vi "Scan Engine.vi"(6 "Message Packet":T1={"Message"="Init", "Parameter"=variant}, 8 "Error In":errorcluster) -> (0 "Error Out":errorcluster)   [LabVIEW 2018]
uses:
  Controls/MessagePacket.ctl
  Controls/QueueNames.ctl
  Controls/Queue Manager Actions.ctl
  Controls/Go Scan Actions.ctl
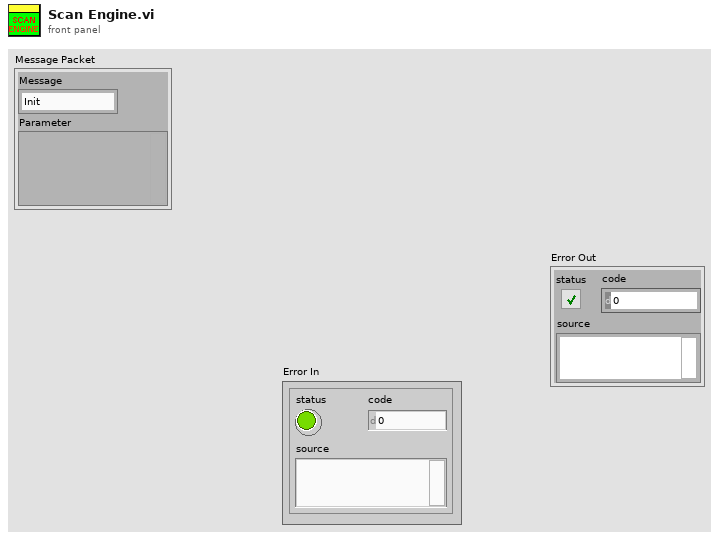
[diagram p1: front panel]
types:
  T1 = typedef "MessagePacket.ctl" = cluster{"Message":string, "Parameter":variant}
  T2 = typedef "Queue Manager Actions.ctl" = enum16{"Init", "Enqueue", "Enqueue All", "Preview Queue", "Dequeue", "Get Status", "Flush Queue", "Flush All Queues", "Release All Queues", "Release Queue", "Enqueue at Opposite End"}
  T3 = typedef "QueueNames.ctl" = enum16{"Main GUI", "Main Scan Processor", "Main Processing", "Main Saving", "Main Display", "Main Table Stage GUI", "Main Table Stage Proc.", "Scan Engine", "Vibratome GUI", "Vibratome Processor", "Slice Engine"}
  T4 = typedef "Go Scan Actions.ctl" = enum16{"Init(ThorOCT Spatial)", "Init(ThorOCT Spectral)", "Init(GPU FFT)", "Init(Alazar FFT)", "Init Scan Head(ThorOCT Spectral)", "Init Scan Head(ThorOCT Spatial)", "Init Scan Head", "Init Table Stage", "Init Vibratome", "Generate Mosaic", "Generate Z Position", "Go to Image Z", "Go Image Home", "Go Mosaic", "Acquire Image(ThorOCT Spatial)", "Acquire Image(ThorOCT Spectral)", "Acquire Image(GPU FFT)", "Acquire Image(Alazar FFT)", "Go Vibratome", "Slice", "Finished(ThorOCT)", "Finished", "Init(Alazar Spectral)"}
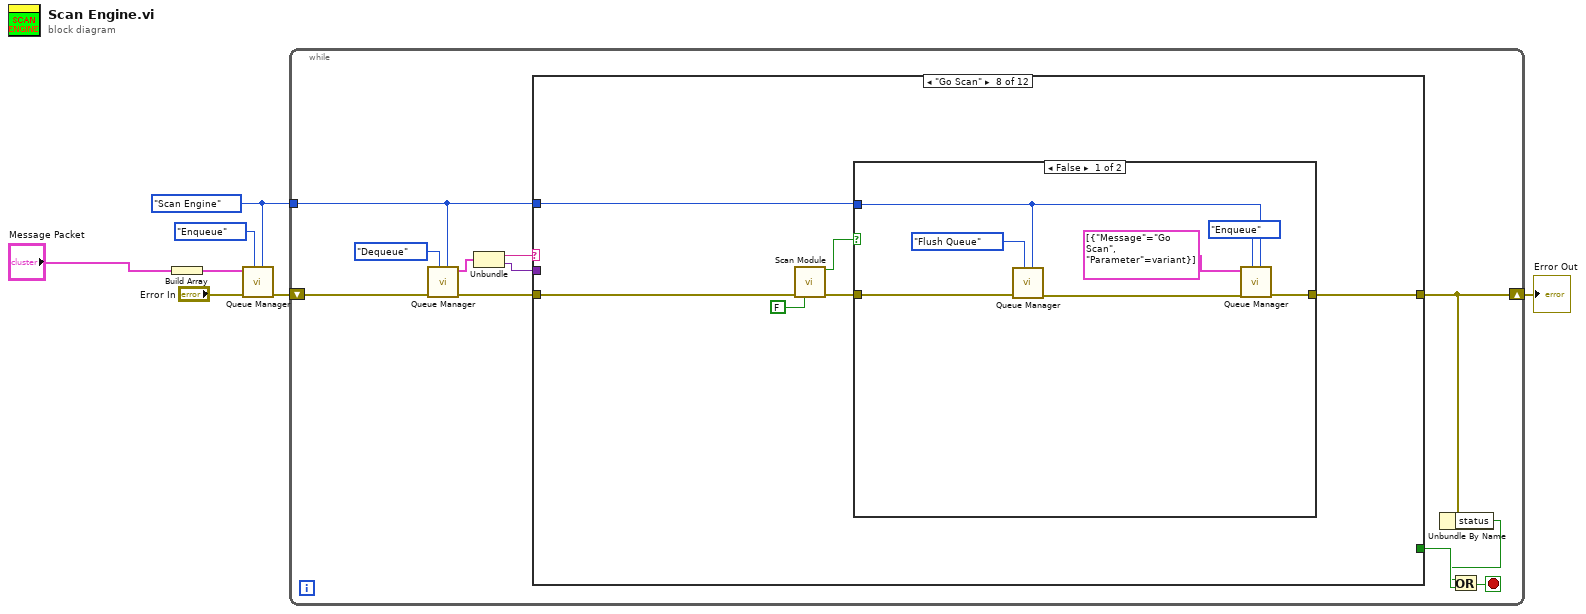
[diagram p0: block diagram]
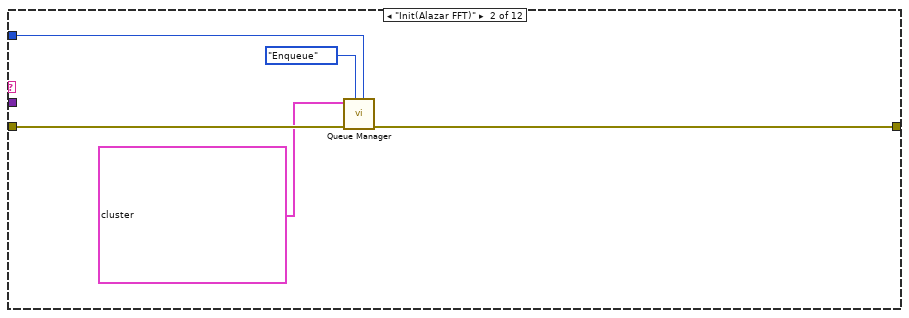
[diagram p3: hidden frame]
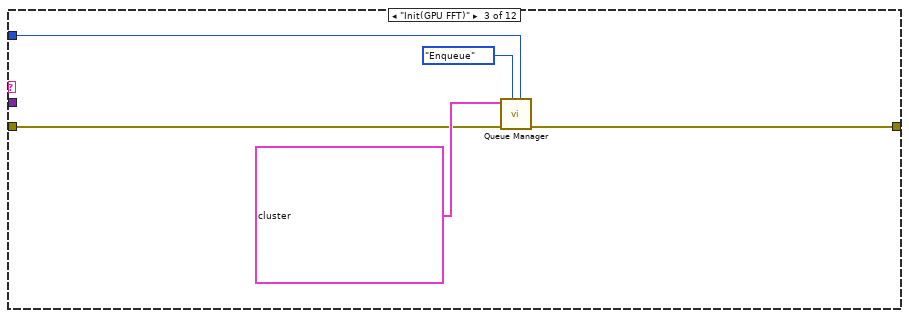
[diagram p4: hidden frame]
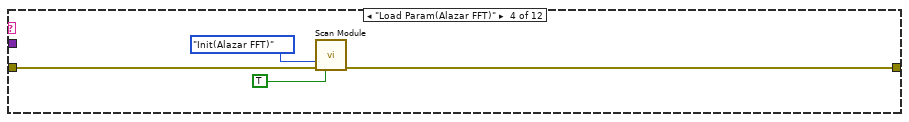
[diagram p5: hidden frame]
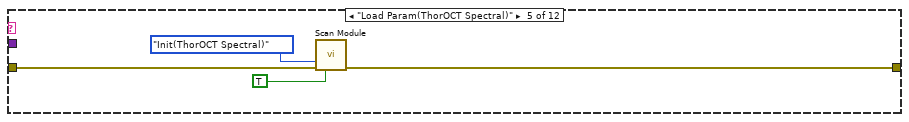
[diagram p6: hidden frame]
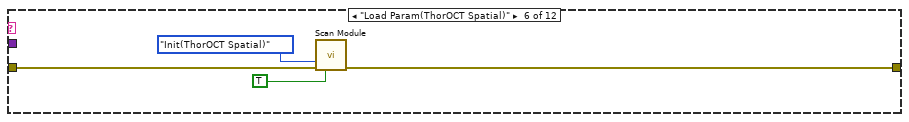
[diagram p7: hidden frame]
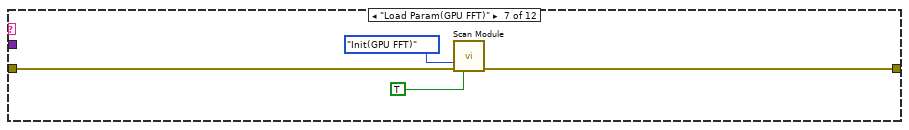
[diagram p8: hidden frame]
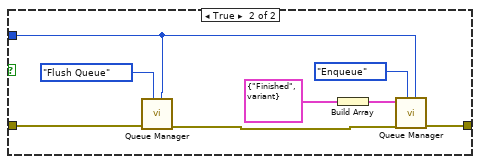
[diagram p9: hidden frame]
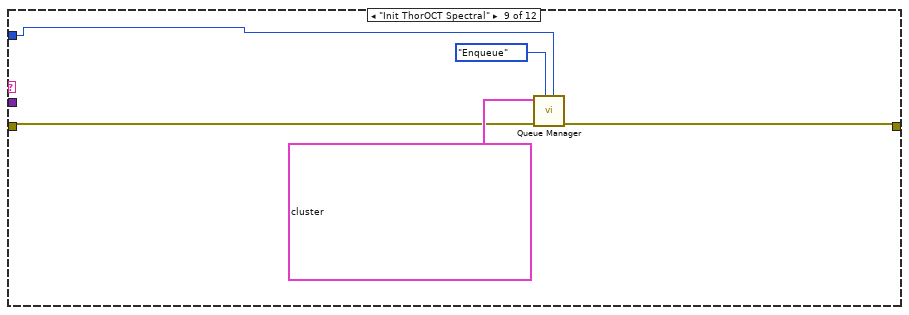
[diagram p10: hidden frame]
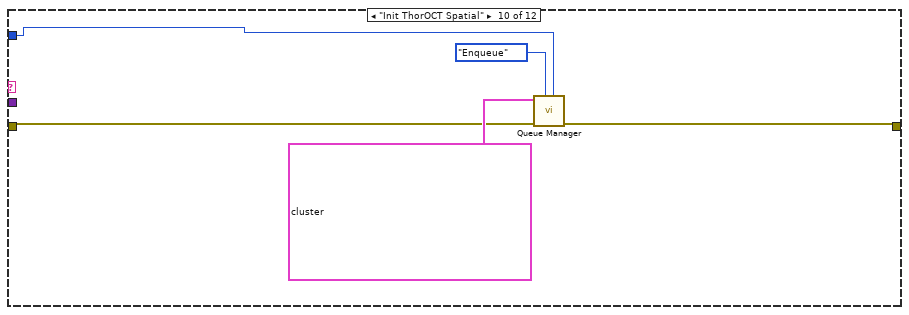
[diagram p11: hidden frame]
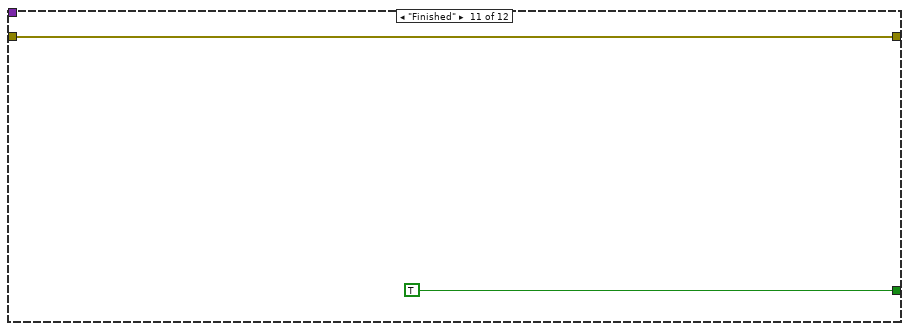
[diagram p12: hidden frame]
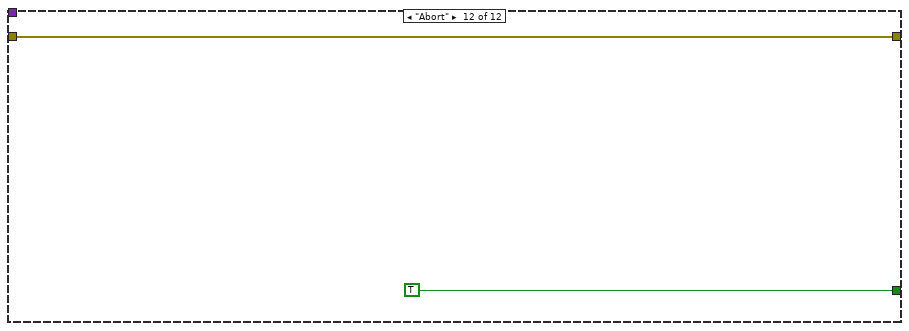
[diagram p13: hidden frame]
diagram:
  w2 = QueueNames."Scan Engine" ("Queue Name")
  n1 = Build Array("Message Packet") -> (w3:T1[])
  n2 = call "Queue Manager.vi"("Queue Name"=w2, "Action"=Queue_Manager_Actions."Enqueue", "Error In"="Error In", "Message Packet Array"=w3) -> ("Error Out"=w5:errorcluster)  [unwired: 3 in, 4 out]
  n3 = while {
    tunnel: w2 -> [w12]
    shift-right: [w9] -> w1
    shift-left: w5 -> [w18]
    stop <- w11 stop-if-true
    n4 = call "Queue Manager.vi"("Queue Name"=w12, "Action"=Queue_Manager_Actions."Dequeue", "Error In"=w18) -> ("Error Out"=w13:errorcluster, "Message Packet [Out]"=w16:T1)  [unwired: 4 in, 3 out]
    n5 = Unbundle(w16) -> ("Message"=w15:string, "Parameter"=w14:variant)
    n6 = case shown="\"Go Scan\"" w15 {
      tunnel: [_ _ _ _ _ _ _ _ _ _ TRUE TRUE] -> w10
      tunnel: w14 -> [_ _ _ _ _ _ _ _ _ _ _ _]
      tunnel: w13 -> [w19 w24 w27 w33 w37 w41 w44 w47 w69 w74 w77 w79]
      tunnel: [w19 w23 w26 w32 w36 w40 w43 w50 w68 w73 w77 w79] -> w9
      tunnel: w12 -> [_ w22 w25 _ _ _ _ w49 w67 w72 _ _]
      frame "Error", Default {
      }
      frame "Init(Alazar FFT)" {
        n7 = call "Queue Manager.vi"("Queue Name"=w22, "Action"=Queue_Manager_Actions."Enqueue", "Error In"=w24, "Message Packet Array"=T1[] [{"Message"="Load Param(Alazar FFT)", "Parameter"=variant}, {"Message"="Go Scan", "Parameter"=variant}]) -> ("Error Out"=w23:errorcluster)  [unwired: 3 in, 4 out]
      }
      frame "Init(GPU FFT)" {
        n8 = call "Queue Manager.vi"("Queue Name"=w25, "Action"=Queue_Manager_Actions."Enqueue", "Error In"=w27, "Message Packet Array"=T1[] [{"Message"="Load Param(GPU FFT)", "Parameter"=variant}, {"Message"="Go Scan", "Parameter"=variant}]) -> ("Error Out"=w26:errorcluster)  [unwired: 3 in, 4 out]
      }
      frame "Load Param(Alazar FFT)" {
        n9 = call "Scan Module.vi"("Init state"=Go_Scan_Actions."Init(Alazar FFT)", "Error In"=w33, "Start Acquire?"=TRUE ("Init")) -> ("Error Out"=w32:errorcluster)  [unwired: 11 in, 1 out]
      }
      frame "Load Param(ThorOCT Spectral)" {
        n10 = call "Scan Module.vi"("Init state"=Go_Scan_Actions."Init(ThorOCT Spectral)", "Error In"=w37, "Start Acquire?"=TRUE ("Init")) -> ("Error Out"=w36:errorcluster)  [unwired: 11 in, 1 out]
      }
      frame "Load Param(ThorOCT Spatial)" {
        n11 = call "Scan Module.vi"("Init state"=Go_Scan_Actions."Init(ThorOCT Spatial)", "Error In"=w41, "Start Acquire?"=TRUE ("Init")) -> ("Error Out"=w40:errorcluster)  [unwired: 11 in, 1 out]
      }
      frame "Load Param(GPU FFT)" {
        n12 = call "Scan Module.vi"("Init state"=Go_Scan_Actions."Init(GPU FFT)", "Error In"=w44, "Start Acquire?"=TRUE ("Init")) -> ("Error Out"=w43:errorcluster)  [unwired: 11 in, 1 out]
      }
      frame "Go Scan" {
        n13 = call "Scan Module.vi"("Error In"=w47, "Start Acquire?"=FALSE) -> ("Finished?"=w51:bool, "Error Out"=w48:errorcluster)  [unwired: 12 in]
        n14 = case shown="False" w51 {
          tunnel: w48 -> [w55 w61]
          tunnel: [w58 w66] -> w50
          tunnel: w49 -> [w52 w59]
          frame False {
            n15 = call "Queue Manager.vi"("Queue Name"=w52, "Action"=Queue_Manager_Actions."Flush Queue", "Error In"=w55) -> ("Error Out"=w54:errorcluster)  [unwired: 4 in, 4 out]
            n16 = call "Queue Manager.vi"("Queue Name"=w52, "Action"=Queue_Manager_Actions."Enqueue", "Error In"=w54, "Message Packet Array"=T1[] [{"Message"="Go Scan", "Parameter"=variant}]) -> ("Error Out"=w58:errorcluster)  [unwired: 3 in, 4 out]
          }
          frame True {
            n17 = call "Queue Manager.vi"("Queue Name"=w59, "Action"=Queue_Manager_Actions."Flush Queue", "Error In"=w61) -> ("Error Out"=w60:errorcluster)  [unwired: 4 in, 4 out]
            n18 = Build Array(T1 {"Message"="Finished", "Parameter"=variant} ("Message Packet")) -> (w63:T1[])
            n19 = call "Queue Manager.vi"("Queue Name"=w59, "Action"=Queue_Manager_Actions."Enqueue", "Error In"=w60, "Message Packet Array"=w63) -> ("Error Out"=w66:errorcluster)  [unwired: 3 in, 4 out]
          }
        }
      }
      frame "Init ThorOCT Spectral" {
        n20 = call "Queue Manager.vi"("Queue Name"=w67, "Action"=Queue_Manager_Actions."Enqueue", "Error In"=w69, "Message Packet Array"=T1[] [{"Message"="Load Param(ThorOCT Spectral)", "Parameter"=variant}, {"Message"="Go Scan", "Parameter"=variant}]) -> ("Error Out"=w68:errorcluster)  [unwired: 3 in, 4 out]
      }
      frame "Init ThorOCT Spatial" {
        n21 = call "Queue Manager.vi"("Queue Name"=w72, "Action"=Queue_Manager_Actions."Enqueue", "Error In"=w74, "Message Packet Array"=T1[] [{"Message"="Load Param(ThorOCT Spatial)", "Parameter"=variant}, {"Message"="Go Scan", "Parameter"=variant}]) -> ("Error Out"=w73:errorcluster)  [unwired: 3 in, 4 out]
      }
      frame "Finished" {
      }
      frame "Abort" {
      }
    }
    n22 = Unbundle By Name(w9) -> ("status"=w8:bool)
    n23 = Or(x=w8, y=w10) -> (x .or. y?=w11:bool)
  }
  "Error Out" <- w1
